vi "TimeStamped CSV File Creation.vi"(10 "Name Convention":string="FP 300MHz and WM 01", 11 "Save Directory":path=path "C:/Users/LabUser/Google Drive/Measurements/11-2017") -> (0 "error out":errorcluster, 3 "path":path)   [LabVIEW 2018]
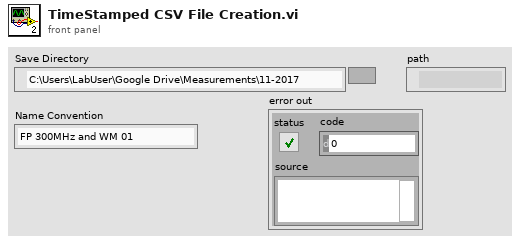
[diagram p1: front panel]
types:
  T1 = enum16{"open", "replace", "create", "open or create", "replace or create", "replace or create with confirmation"}
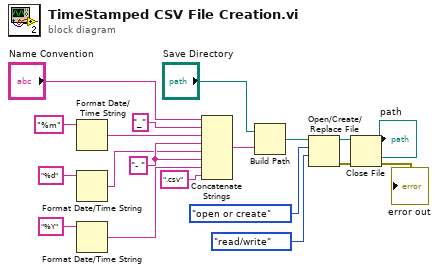
[diagram p0: block diagram]
diagram:
  w18 = "- " ("string")
  n1 = Format Date/Time String(time format string (%c)="%m") -> (date/time string=w12:string)  [unwired: 2 in]
  n2 = Format Date/Time String(time format string (%c)="%d") -> (date/time string=w5:string)  [unwired: 2 in]
  n3 = Format Date/Time String(time format string (%c)="%Y") -> (date/time string=w6:string)  [unwired: 2 in]
  n4 = Concatenate Strings("Name Convention", "_" ("string"), w12, w18, w5, w18, w6, ".csv" ("string")) -> (w14:string)
  n5 = Build Path(base path="Save Directory", name or relative path=w14) -> (appended path=w7:path)
  n6 = Open/Create/Replace File(file path (use dialog)=w7, operation (0:open)=T1."open or create", access (0:read/write)=enum16{"read/write", "read-only", "write-only"}."read/write") -> (refnum out=w11:refnum<file>, error out=w10:errorcluster)  [unwired: 3 in, 1 out]
  n7 = Close File(refnum=w11, error in=w10) -> (path=→"path":path, error out=→"error out":errorcluster)
